vi "Construct Controller.vi"(8 "error in (no error)":errorcluster, 10 "TCP Timeout":i32, 11 "TCP Port":u16) -> (0 "error out":errorcluster, 3 "tWorkerController out":refnum<class "tWorkerController.lvclass">)   [LabVIEW 2013, in "tWorkerController.lvlib" / "tWorkerController.lvclass"]
uses:
  tWorkerController.lvclass
  tWorkerController.lvclass/tWorkerController.ctl
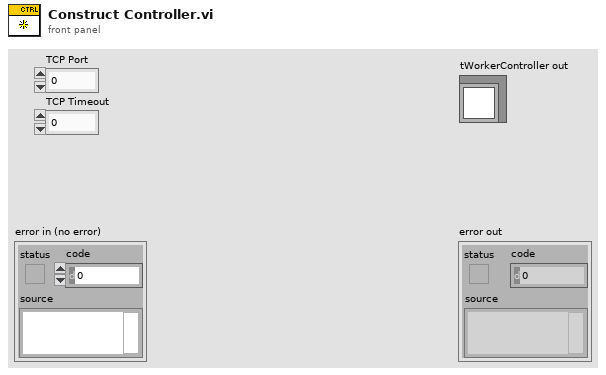
[diagram p1: front panel]
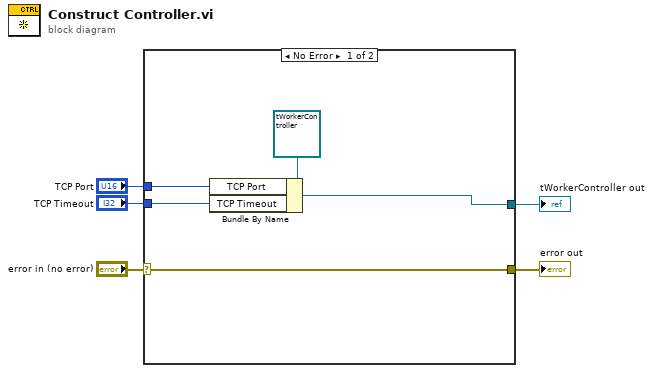
[diagram p0: block diagram]
diagram:
  n1 = case shown="No Error" "error in (no error)" {
    selector: "error in (no error)" -> [w6 w11]
    tunnel: [w6 w11] -> w4
    tunnel: "TCP Port" -> [w9 _]
    tunnel: "TCP Timeout" -> [w8 _]
    tunnel: [w7 _] -> w1
    frame No Error {
      n2 = Bundle By Name(cluster=refnum<class "tWorkerController.lvclass"> refnum ("tWorkerController out"), "TCP Port"=w9, "TCP Timeout"=w8) -> (w7:refnum<class "tWorkerController.lvclass">)
    }
    frame Error {
    }
  }
  "error out" <- w4
  "tWorkerController out" <- w1
